vi "Get Actor Handles.vi"() -> (2 "Actor Handles":refnum<class "Protected Actor Handle.lvclass">[](array[class]))   [LabVIEW 2025, in "AF Debug.lvlib"]
doc: "This VI returns an array of handles for currently running actors to use in a debugging tool. Actors are wrapped in handles to limit a debugger's ability to interfere with the operation of the actors and to protect the debugger from actors stopping unexpectedly.\n\nThis VI is a wrapper for a VI of the same name in Actor Framework.lvlib. It has been provided to support tools written to use older versions of the AF Debug library. It is DEPRECATED, but functional."
uses:
  AF Debug.lvlib
  Protected Actor Handle/Protected Actor Handle.lvclass
  vi.lib/ActorFramework/Actor Framework.lvlib
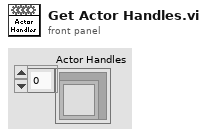
[diagram p1: front panel]
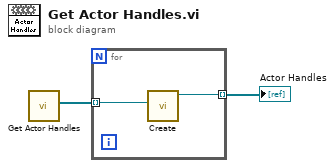
[diagram p0: block diagram]
diagram:
  n1 = call "Get Actor Handles.vi"() -> ("Actor Handles"=w2:refnum<class "Protected Actor Handle.lvclass">[])  [unwired: 11 in]
  n2 = for {
    tunnel: w2 -> [w4] mode=indexing
    tunnel: [w3] -> w1 mode=indexing
    n3 = call "Create.vi"("Handle"=w4) -> ("Protected Actor Handle out"=w3:refnum<class "Protected Actor Handle.lvclass">)  [unwired: 9 in, 1 out]
  }
  "Actor Handles" <- w1
